vi "CRYSet Replace File Front Panel.vi"(11 "Vi Ref":refnum<vi>) -> ()   [LabVIEW 2013]
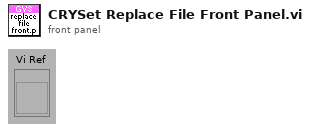
[diagram p1: front panel]
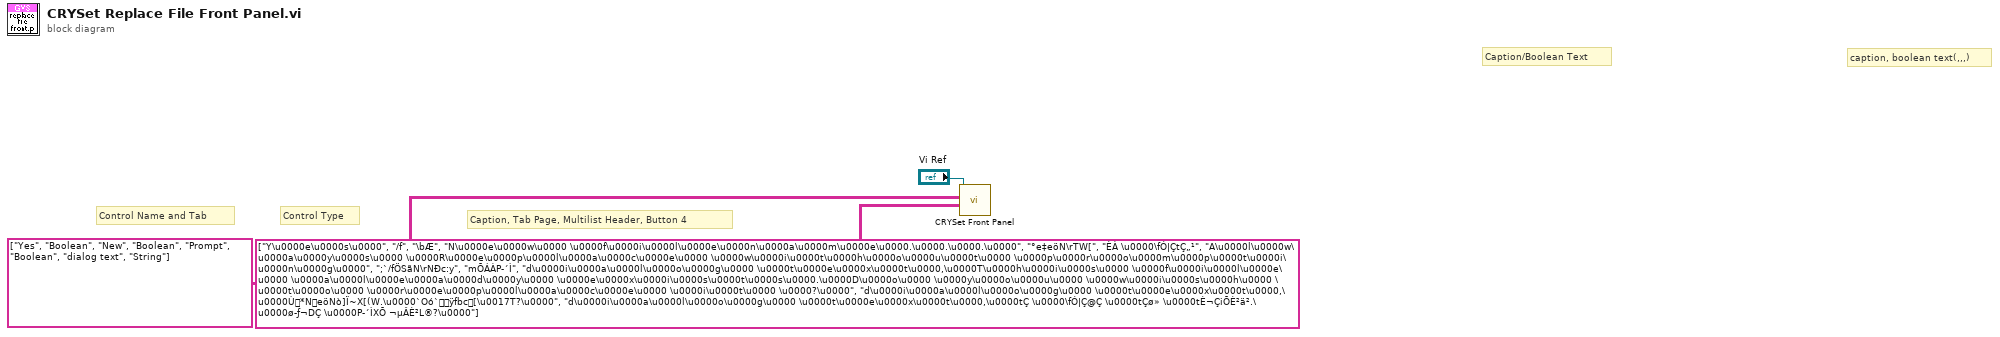
[diagram p0: block diagram]
diagram:
  # "Caption, Tab Page, Multilist Header, Button 4"
  # "Control Type"
  # "Control Name and Tab"
  # "caption, boolean text(,,,)"
  # "Caption/Boolean Text"
  n1 = call "CRYSet Front Panel.vi"("Caption(Boolean Text)"=string[][] [["Y\u0000e\u0000s\u0000", "/f", "\bÆ"], ["N\u0000e\u0000w\u0000 \u0000f\u0000i\u0000l\u0000e\u0000n\u0000a\u0000m\u0000e\u0000.\u0000.\u0000.\u0000", "°e‡eöN\rTW[", "ÈÀ \u0000\fÓ|ÇtÇ„¹"], ["A\u0000l\u0000w\u0000a\u0000y\u0000s\u0000 \u0000R\u0000e\u0000p\u0000l\u0000a\u0000c\u0000e\u0000 \u0000w\u0000i\u0000t\u0000h\u0000o\u0000u\u0000t\u0000 \u0000p\u0000r\u0000o\u0000m\u0000p\u0000t\u0000i\u0000n\u0000g\u0000", ";`/fÖSãN\rNÐc:y", "mÕÁÀP­´Ì"], ["d\u0000i\u0000a\u0000l\u0000o\u0000g\u0000 \u0000t\u0000e\u0000x\u0000t\u0000,\u0000T\u0000h\u0000i\u0000s\u0000 \u0000f\u0000i\u0000l\u0000e\u0000 \u0000a\u0000l\u0000e\u0000a\u0000d\u0000y\u0000 \u0000e\u0000x\u0000i\u0000s\u0000t\u0000s\u0000.\u0000D\u0000o\u0000 \u0000y\u0000o\u0000u\u0000 \u0000w\u0000i\u0000s\u0000h\u0000 \u0000t\u0000o\u0000 \u0000r\u0000e\u0000p\u0000l\u0000a\u0000c\u0000e\u0000 \u0000i\u0000t\u0000 \u0000?\u0000", "d\u0000i\u0000a\u0000l\u0000o\u0000g\u0000 \u0000t\u0000e\u0000x\u0000t\u0000,\u0000Ù*NeöNò]Ï~X[(W.\u0000`Oó`ÿfbc[\u0017T?\u0000", "d\u0000i\u0000a\u0000l\u0000o\u0000g\u0000 \u0000t\u0000e\u0000x\u0000t\u0000,\u0000tÇ \u0000\fÓ|Ç@Ç \u0000tÇø» \u0000tÈ¬ÇiÕÈ²ä².\u0000ø­ƒ¬DÇ \u0000P­´ÌXÕ ¬µÂÈ²L®?\u0000"]], "Control ID and Type(Label Name, Type)"=string[][] [["Yes", "Boolean"], ["New", "Boolean"], ["Prompt", "Boolean"], ["dialog text", "String"]], "Vi Ref"="Vi Ref") -> ()  [unwired: 9 in]
